vi "Write XML file.vi"(8 "error in (no error)":errorcluster, 10 "Array in":string[](array[string]), 11 "file path (use dialog)":path) -> (0 "error out":errorcluster, 2 "xml string":string, 3 "path":path)   [LabVIEW 2012]
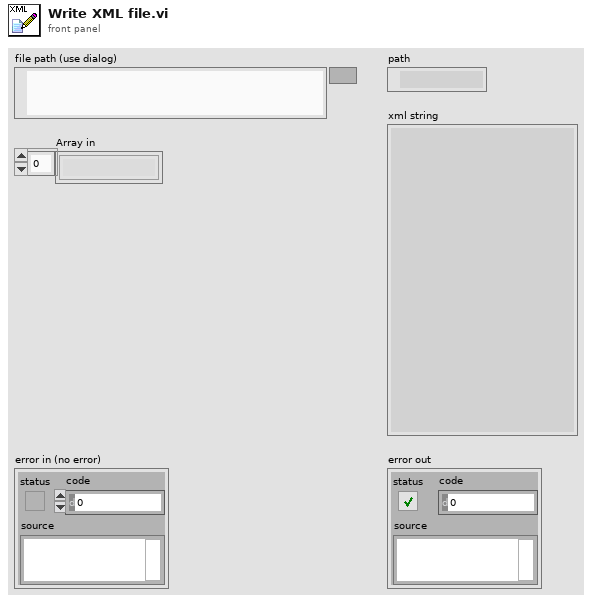
[diagram p1: front panel]
types:
  T1 = enum16{"open", "replace", "create", "open or create", "replace or create", "replace or create with confirmation"}
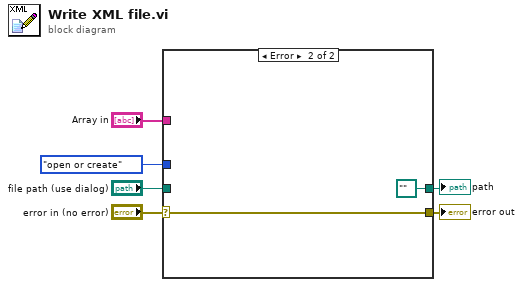
[diagram p0: block diagram]
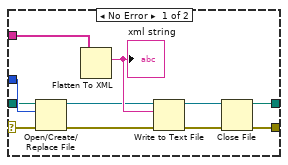
[diagram p2: hidden frame]
diagram:
  n1 = case shown="Error" "error in (no error)" {
    selector: "error in (no error)" -> [w7 w18]
    tunnel: [w17 path "" ("path")] -> w6
    tunnel: [w16 w18] -> w5
    tunnel: "Array in" -> [w15 _]
    tunnel: T1."open or create" ("operation (0:open)") -> [w9 _]
    tunnel: "file path (use dialog)" -> [w8 _]
    frame No Error {
      n2 = Open/Create/Replace File(file path (use dialog)=w8, error in=w7, operation (0:open)=w9) -> (refnum out=w10:refnum<file>, error out=w11:errorcluster)  [unwired: 3 in, 1 out]
      n3 = Flatten To XML(anything=w15) -> (xml string=w14:string)
      "xml string" <- w14
      n4 = Write to Text File(file (use dialog)=w10, text=w14, error in=w11) -> (refnum out=w12:refnum<file>, error out=w13:errorcluster)  [unwired: 1 in, 1 out]
      n5 = Close File(refnum=w12, error in=w13) -> (path=w17:path, error out=w16:errorcluster)
    }
    frame Error {
    }
  }
  "error out" <- w5
  "path" <- w6
